vi "uTransport_Queue_Create.vi"(8 "error in (no error)":errorcluster) -> (0 "error out":errorcluster, 2 "queue":refnum<queue>, 3 "uTransport_Queue out":refnum<class "uTransport_Queue.lvclass">)   [LabVIEW 2023, in "uLib.lvlib" / "uTransport_Queue.lvclass"]
doc: "Do NOT do a LV native 'release queue'. Use the Destroy method instead."
uses:
  uTransport_Queue.lvclass
  uMsg/uMsg/uMsg.lvclass
  uTransport_Queue.lvclass/uTransport_Queue.ctl
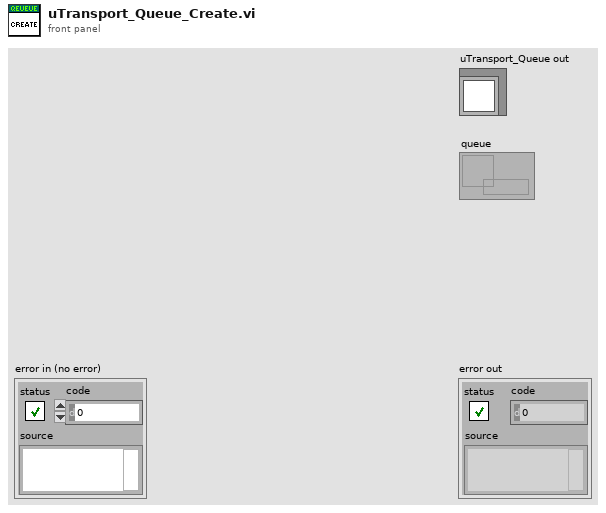
[diagram p1: front panel]
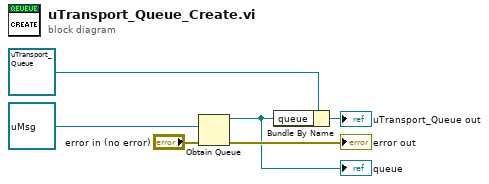
[diagram p0: block diagram]
diagram:
  n1 = Obtain Queue(element data type=refnum<class "uMsg.lvclass"> refnum ("uTransport.lvlib:uMsg.lvclass"), error in (no error)="error in (no error)") -> (queue out=w1:refnum<queue>, error out=→"error out":errorcluster)  [unwired: 3 in, 1 out]
  "queue" <- w1
  n2 = Bundle By Name(cluster=refnum<class "uTransport_Queue.lvclass"> refnum ("uTransport_Queue out"), "queue"=w1) -> (→"uTransport_Queue out":refnum<class "uTransport_Queue.lvclass">)
